vi "Pre Launch Init.vi"(11 "User Interface in":refnum<class "User Interface.lvclass">) -> (0 "error out":errorcluster, 3 "User Interface out":refnum<class "User Interface.lvclass">)   [LabVIEW 2016, in "User Interface.lvlib" / "User Interface.lvclass"]
doc: "(<B>Filename</B>: Actor Framework.lvlib:Actor.lvclass:Pre Launch Init.vi)\n\nDefines behavior that occurs after the Launch Nested Actor method is invoked but before the actor's Actor Core method begins running.\n\nBy default, this method does nothing. A descendant class may override it to define behavior."
uses:
  User Interface.lvclass
  Configurations/Configurations.lvclass
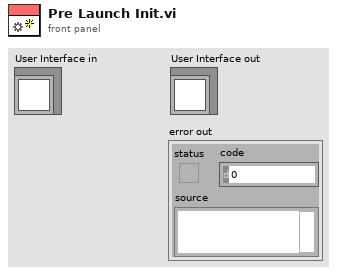
[diagram p1: front panel]
types:
  T1 = typedef "Configurations.lvlib/Configurations.lvclass/Session Handle.ctl" = refnum<data-value>
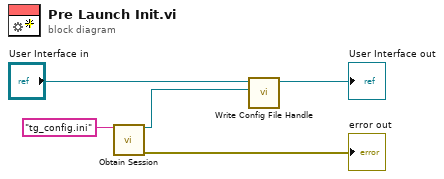
[diagram p0: block diagram]
diagram:
  n1 = call "Obtain Session.vi"("Filename"="tg_config.ini") -> ("Session Handle"=w1:T1, "error out"=→"error out":errorcluster)  [unwired: 13 in]
  n2 = call-dynamic "Write Config File Handle.vi"("Session Handle"=w1, "User Interface in"="User Interface in") -> ("User Interface out"=→"User Interface out":refnum<class "User Interface.lvclass">)  [unwired: 9 in]
